vi "Concatenate State with Arguments.vi"(10 "Arguments":string, 11 "State":string) -> (3 "State with Arguements":string)   [LabVIEW 2020, in "Communicable State Machine.lvlib"]
uses:
  Communicable State Machine.lvlib
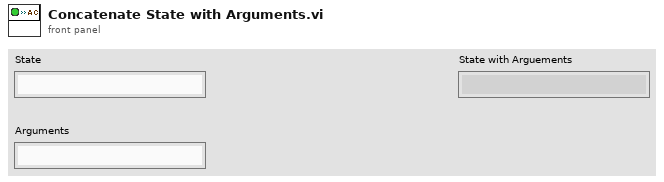
[diagram p1: front panel]
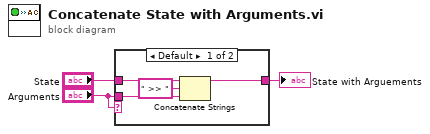
[diagram p0: block diagram]
diagram:
  n1 = case "Is arguments empty? If so, then do not append arguments" shown="Default" "Arguments" {
    tunnel: [w4 w8] -> w3
    tunnel: "State" -> [w7 w8]
    tunnel: "Arguments" -> [w5 _]
    frame Default {
      n2 = Concatenate Strings(w7, " >> " ("string"), w5) -> (w4:string)
    }
    frame "" {
    }
  }
  "State with Arguements" <- w3
